vi "Example - Single On-Off.vi"() -> ()   [LabVIEW 2017]
uses:
  Power Supply_class/Power Supply.lvclass
panel:
  in  "Power Supply Chain Address":i16=1
  in  "Set Current (A)":dbl=1.0
  in  "Set Voltage (V)":dbl=5.0
  in  "Open Power Supply":bool
  in  "Quit Program":bool
  in  "Power Supply Chain VISA Resource Name":refnum<visa-resource-name>="COM13"
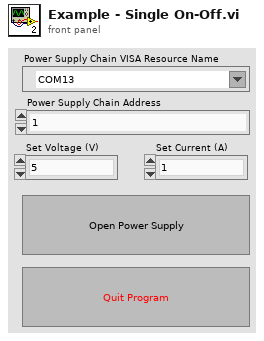
[diagram p1: front panel]
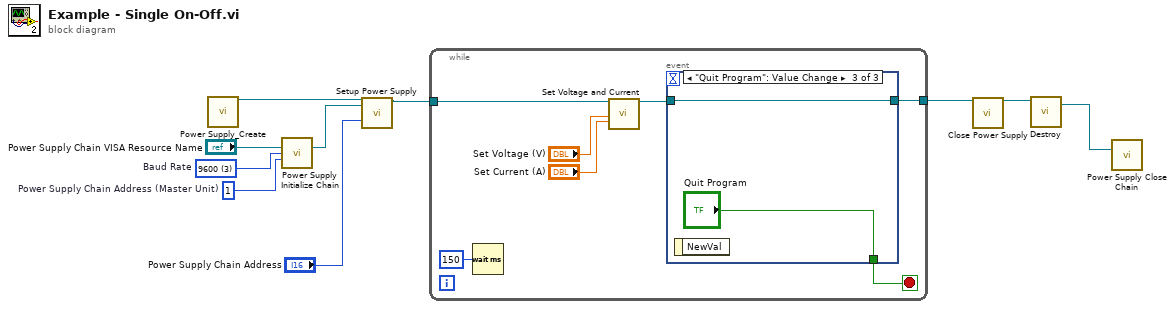
[diagram p0: block diagram]
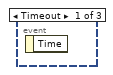
[diagram p2: hidden frame]
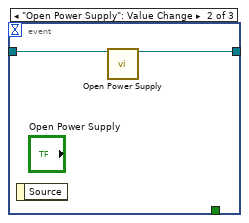
[diagram p3: hidden frame]
diagram:
  w2 = i16 1  # Power Supply Chain Address (Master Unit)
  w7 = u16 3 items=["1200", "2400", "4800", "9600", "19200"]  # Baud Rate
  n1 = call "Power Supply_Create.vi"() -> ("reference out"=w10:refnum<class "Power Supply.lvclass">)  [unwired: 18 in, 1 out]
  n2 = call "Power Supply Initialize Chain.vi"("Power Supply Chain VISA Resource"="Power Supply Chain VISA Resource Name", "Baud Rate"=w7, "Power Supply Chain Address (Master Unit)"=w2) -> ("PowerSupply Chain VISA Session"=w9:refnum<visa-resource-name>)  [unwired: 10 in, 2 out]
  n3 = call-dynamic "Setup Power Supply.vi"("reference in"=w10, "Power Supply Chain VISA Session"=w9, "Power Supply Chain Address"="Power Supply Chain Address") -> ("reference out"=w3:refnum<class "Power Supply.lvclass">)  [unwired: 14 in, 2 out]
  n4 = while {
    tunnel: [w16] -> w4
    tunnel: w3 -> [w12]
    stop <- w17 stop-if-true
    n5 = Wait (ms)(milliseconds to wait=u32 150) -> ()  [unwired: 1 out]
    n6 = call-dynamic "Set Voltage and Current.vi"("reference in"=w12, "Set Voltage (V)"="Set Voltage (V)", "Set Current (A)"="Set Current (A)") -> ("reference out"=w11:refnum<class "Power Supply.lvclass">)  [unwired: 15 in, 1 out]
    n7 = event shown="[2] \"Quit Program\": Value Change" {
      selector: _ -> [_ _ _]
      dyn-events: _ -> [_ _ _]
      timeout: _ -> [_ _ _]
      tunnel: [_ _ "Quit Program"] -> w17
      tunnel: w11 -> [_ w19 w20]
      tunnel: [_ w18 w20] -> w16
      event Timeout {
        n8 = event-data() -> ()  [unwired: 1 in, 1 out]
      }
      event "Open Power Supply": Value Change {
        n9 = event-data() -> ()  [unwired: 1 in, 1 out]
        n10 = call-dynamic "Open Power Supply.vi"("reference in"=w19) -> ("reference out"=w18:refnum<class "Power Supply.lvclass">)  [unwired: 16 in, 2 out]
      }
      event "Quit Program": Value Change {
        n11 = event-data() -> ()  [unwired: 1 in, 1 out]
      }
    }
  }
  n12 = call-dynamic "Close Power Supply.vi"("reference in"=w4) -> ("reference out"=w5:refnum<class "Power Supply.lvclass">)  [unwired: 16 in, 2 out]
  n13 = call-dynamic "Destroy.vi"("reference in"=w5) -> ("Power Supply Chain VISA Session"=w6:refnum<visa-resource-name>)  [unwired: 16 in, 2 out]
  n14 = call "Power Supply Close Chain.vi"("Power Supply Chain VISA Session"=w6) -> ()  [unwired: 14 in, 1 out]
